vi "Teststand Edit STP.vi"(8 "error in":errorcluster, 10 "STP Data in":T1={"ECU CAN Port"="CAN1", "CMD"=130, "CAN Write Data"=[], "Response Decoder"=enum."String", "String"={"Start Index"=0, "Length"=-1}, "Number"={"MSB Index"=0, "LSB Index"=1}, "Boolean"={"Index"=0, "Bool"={"7"=FALSE, "6"=FALSE, "5"=FALSE, "4"=FALSE, "3"=FALSE, "2"=FALSE, "1"=FALSE, "0"=FALSE, "7 Enabled"=FALSE, "6 Enabled"=FALSE, "5 Enabled"=FALSE, "4 Enabled"=FALSE, "3 Enabled"=FALSE, "2 Enabled"=FALSE, "1 Enabled"=FALSE, "0 Enabled"=FALSE}}} {"CMD" items=["TSW_VERSION(130)"=130, "WAIT_EVENT(132)"=132, "SEQUENCER(133)"=133, "TSW_RESET(150)"=150, "CONFIG_ECU(151)"=151, "TEST_CORE (152)"=152, "TEST_WATCHDOG (153)"=153, "TEST_MONITORING (154)"=154, "READ_MEMORY (162)"=162, "WRITE_ERASE_MEMORY (164)"=164, "COMM_EXTERNAL (190)"=190, "COMM_INTERNAL (195)"=195, "GET_ANALOG_INPUT (210)"=210, "GET_DIGITAL_INPUT (211)"=211, "GET_FREQUENCY_INPUT (212)"=212, "TEST_INPUT_STRUCTURE (214)"=214, "GENERATE_OUTPUT_SIGNAL (220)"=220, "GENERATE_SYNCHRONIZED_OUTPUT_SIGNALS (221)"=221, "eDCU_Specific (250)"=250]; "CAN Write Data" format="%.0x"}, 11 "Sequence Context In":refnum<k7>) -> (0 "error out":errorcluster, 2 "STP Data out":T1={"ECU CAN Port"="CAN1", "CMD"=130, "CAN Write Data"=[], "Response Decoder"=enum."String", "String"={"Start Index"=0, "Length"=-1}, "Number"={"MSB Index"=0, "LSB Index"=1}, "Boolean"={"Index"=0, "Bool"={"7"=FALSE, "6"=FALSE, "5"=FALSE, "4"=FALSE, "3"=FALSE, "2"=FALSE, "1"=FALSE, "0"=FALSE, "7 Enabled"=FALSE, "6 Enabled"=FALSE, "5 Enabled"=FALSE, "4 Enabled"=FALSE, "3 Enabled"=FALSE, "2 Enabled"=FALSE, "1 Enabled"=FALSE, "0 Enabled"=FALSE}}} {"CMD" items=["TSW_VERSION(130)"=130, "WAIT_EVENT(132)"=132, "SEQUENCER(133)"=133, "TSW_RESET(150)"=150, "CONFIG_ECU(151)"=151, "TEST_CORE (152)"=152, "TEST_WATCHDOG (153)"=153, "TEST_MONITORING (154)"=154, "READ_MEMORY (162)"=162, "WRITE_ERASE_MEMORY (164)"=164, "COMM_EXTERNAL (190)"=190, "COMM_INTERNAL (195)"=195, "GET_ANALOG_INPUT (210)"=210, "GET_DIGITAL_INPUT (211)"=211, "GET_FREQUENCY_INPUT (212)"=212, "TEST_INPUT_STRUCTURE (214)"=214, "GENERATE_OUTPUT_SIGNAL (220)"=220, "GENERATE_SYNCHRONIZED_OUTPUT_SIGNALS (221)"=221, "eDCU_Specific (250)"=250]; "CAN Write Data" format="%.0x"})   [LabVIEW 2023, in "LTT_TeststandSteptypes.lvlib"]
uses:
  LTT_TeststandSteptypes.lvlib
  Control/STP Data.ctl
  HardwareAbstractionLayer_LVOOP/CAN/CAN Application Protocols/STP Protocol_class/Ctrls/STP CMD.ctl
  <vilib>/addons/TestStand/_TSUtility.llb/TestStand - Start Modal Dialog (Sequence Context).vi
  <vilib>/addons/TestStand/_TSUtility.llb/TestStand - End Modal Dialog (Sequence Context).vi
  HardwareAbstractionLayer_LVOOP/Database/Database.lvclass
  HardwareAbstractionLayer_LVOOP/Database/SQL Public VI/Control/DB Options.ctl
  HardwareAbstractionLayer_LVOOP/CAN/CAN Application Protocols/STP Protocol_class/STP Protocol.lvclass
panel:
  in  "Close":bool
  in  "OK":bool
  # "Help : the index will choose the one element in an array and compare its true or false"
  # "Bit"
  # "Value"
  # "Enabled"
  # "Help : if the LSB index is -1 then it will take only MSB value"
  # "Help : if length -1 then it will take the entire array"
  # "Help : the index will choose the one element in an array and compare its true or false"
  # "Bit"
  # "Value"
  # "Enabled"
  # "Help : if the LSB index is -1 then it will take only MSB value"
  # "Help : if length -1 then it will take the entire array"
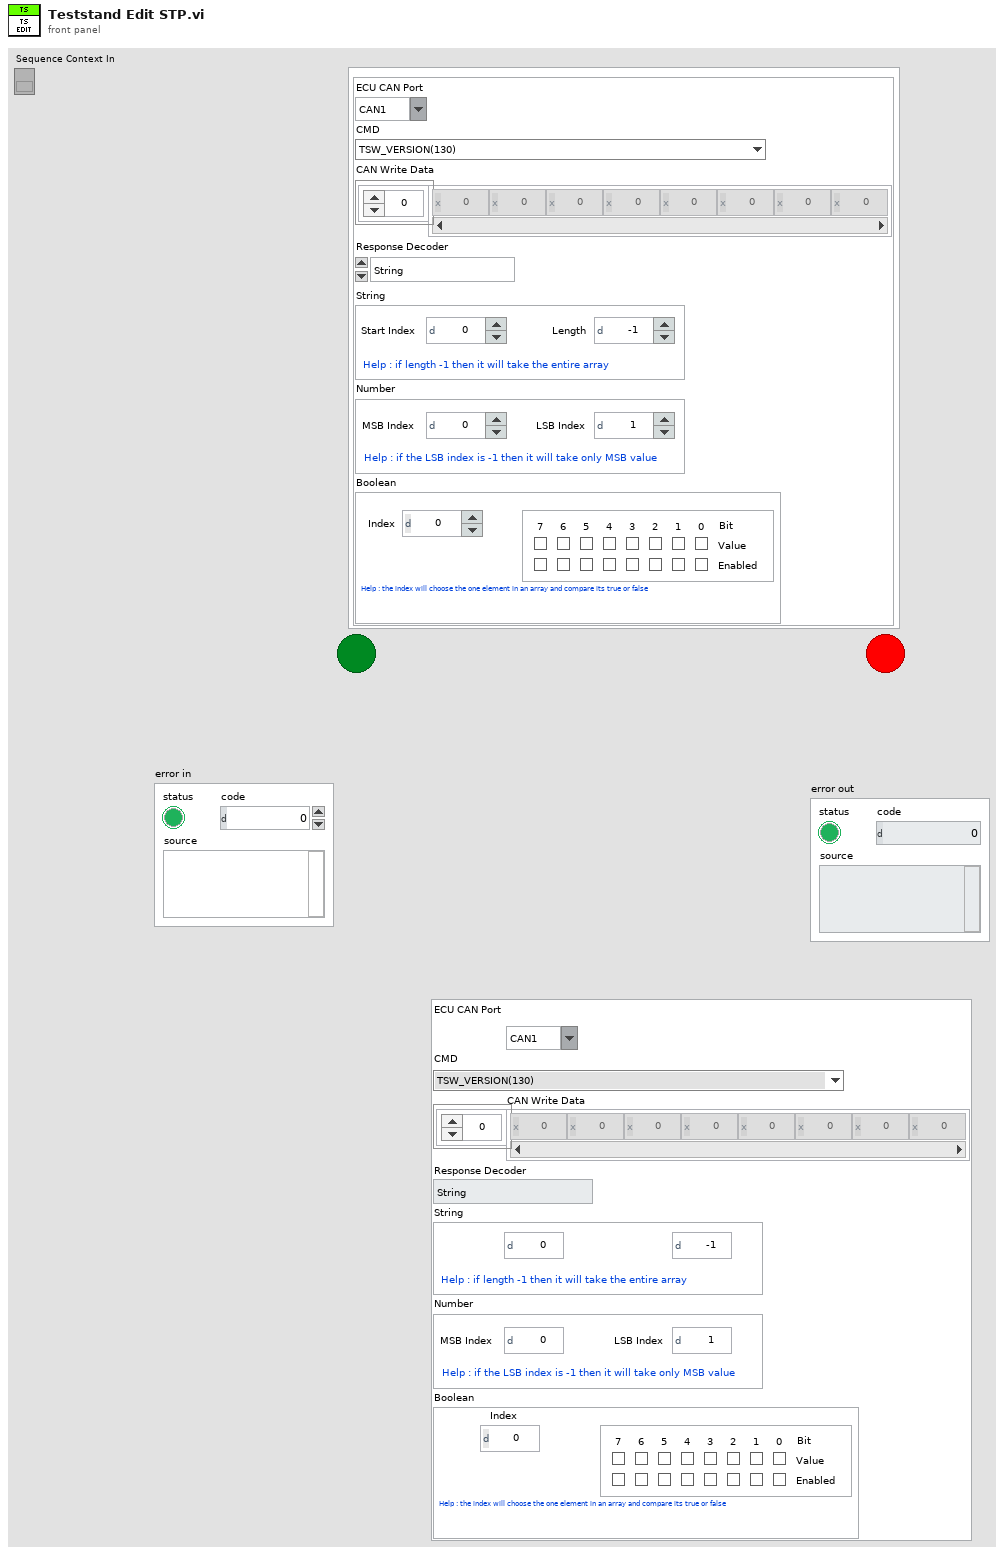
[diagram p1: front panel]
types:
  T1 = typedef "LTT_TeststandSteptypes.lvlib/STP Data.ctl" = cluster{"ECU CAN Port":string, "CMD":T2, "CAN Write Data":u8[], "Response Decoder":enum16{"String", "Number", "Boolean"}, "String":cluster{"Start Index":i32, "Length":i32}, "Number":cluster{"MSB Index":i32, "LSB Index":i32}, "Boolean":cluster{"Index":i32, "Bool":cluster{"7":bool, "6":bool, "5":bool, "4":bool, "3":bool, "2":bool, "1":bool, "0":bool, "7 Enabled":bool, "6 Enabled":bool, "5 Enabled":bool, "4 Enabled":bool, "3 Enabled":bool, "2 Enabled":bool, "1 Enabled":bool, "0 Enabled":bool}}}
  T2 = typedef "HardwareAbstractionLayer_LVOOP.lvlib/CAN Application Protocols Lib.lvlib/STP Protocol.lvclass/STP CMD.ctl" = u8
  T3 = typedef "HardwareAbstractionLayer_LVOOP.lvlib/Database.lvclass/DB Options.ctl" = enum16{"Init", "Select Data", "Insert Data", "Update Data", "Delete Data", "Execute Query", "Create Schema", "Create Table", "List Tables", "List Columns", "Close"}
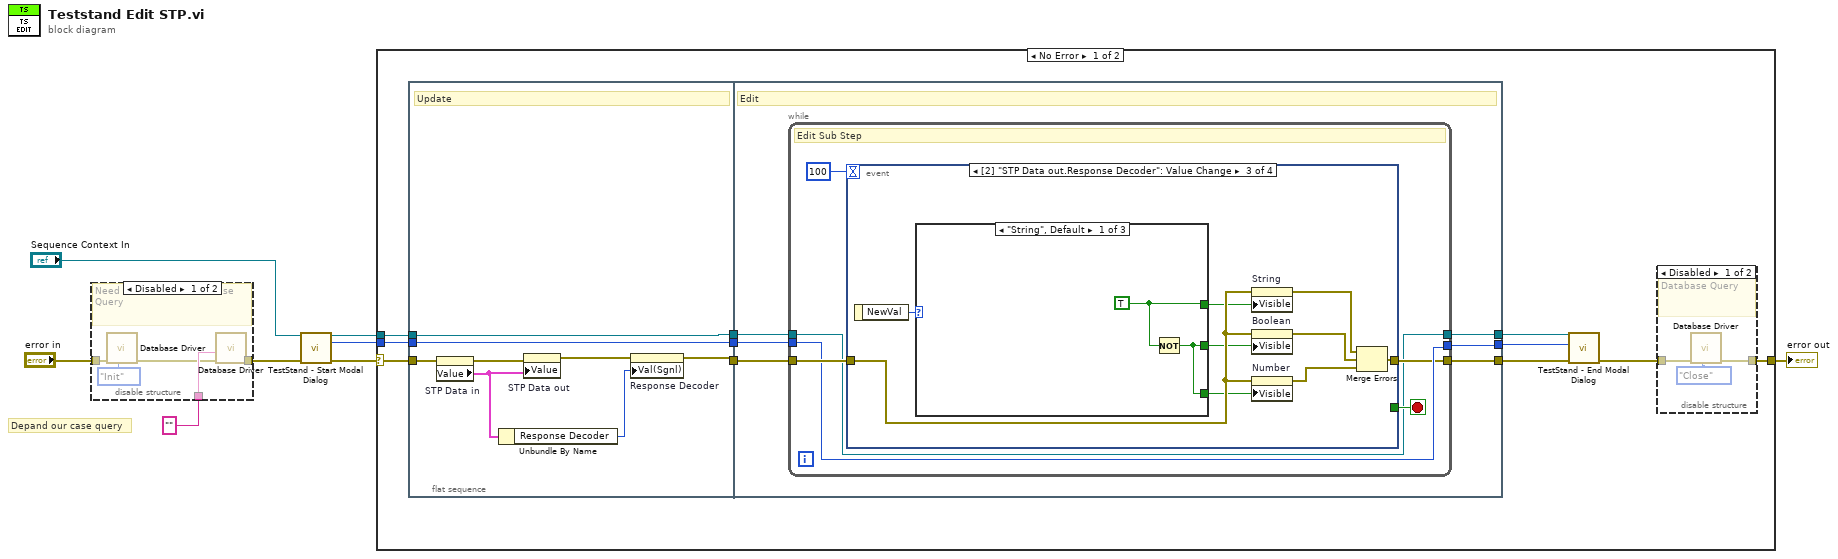
[diagram p0: block diagram]
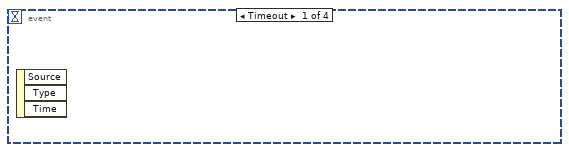
[diagram p3: hidden frame]
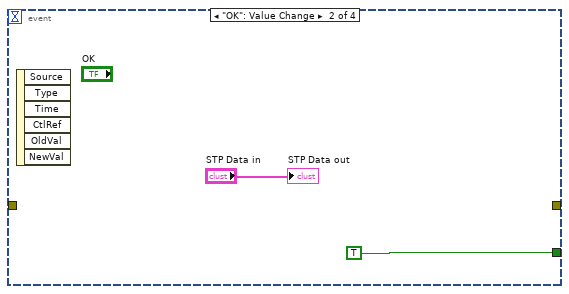
[diagram p4: hidden frame]
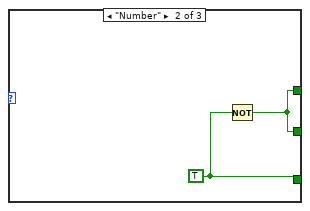
[diagram p5: hidden frame]
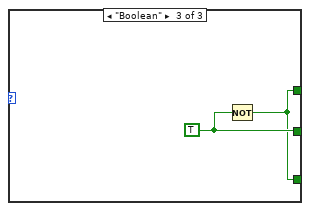
[diagram p6: hidden frame]
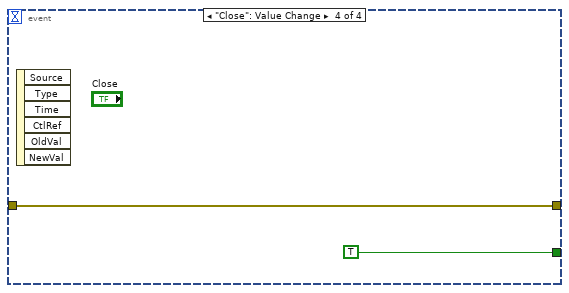
[diagram p7: hidden frame]
diagram:
  # "Depand our case query"
  n1 = disable-structure shown="Disabled" {
    disable-tunnel: "error in" -> [w13 _]
    disable-tunnel: [w12 _] -> w3
    disable-tunnel: "" ("SQL query") -> [w11 _]
    frame Disabled {
      # "Need to Enable for Database Query"
      n2 = call "Database Driver.vi"("Options"=DB_Options."Init", "error in"=w13) -> ("error out"=w10:errorcluster)  [unwired: 6 in, 3 out]
      n3 = call "Database Driver.vi"("error in"=w10, "SQL query"=w11) -> ("error out"=w12:errorcluster)  [unwired: 6 in, 3 out]
    }
    frame Enabled {
    }
  }
  n4 = call-poly <vilib>:"TestStand - Start Modal Dialog.vi"("Sequence Context In"="Sequence Context In", "error in (no error)"=w3) -> ("Sequence Context Out"=w5:refnum<k7>, "Modal ID"=w4:i32, "error out"=w6:errorcluster)  [unwired: 9 in, 2 out]
  n5 = case shown="No Error" w6 {
    selector: w6 -> [w21 w67]
    tunnel: w5 -> [w18 _]
    tunnel: w4 -> [w17 _]
    tunnel: [w15 w67] -> w1
    frame No Error {
      n6 = flat-sequence {
        tunnel: w21 -> [w33]
        tunnel: [w30] -> w24
        tunnel: w18 -> [w35]
        tunnel: w17 -> [w34]
        tunnel: [w35] -> w23
        tunnel: [w34] -> w22
        tunnel: w24 -> [w39]
        tunnel: [w37] -> w20
        tunnel: w23 -> [w41]
        tunnel: w22 -> [w40]
        tunnel: [w38] -> w16
        tunnel: [w36] -> w14
        frame #0 {
          # "Update"
          n7 = property on="STP Data in" class="Clust (strict)"(error in=w33) -> (error out=w32:errorcluster, "Value"=w29:T1)  [unwired: 1 in, 1 out]
          n8 = Unbundle By Name(w29) -> ("Response Decoder"=w28:enum16{"String", "Number", "Boolean"})
          n9 = property on="STP Data out" class="Clust (strict)"(error in=w32, "Value"=w29) -> (error out=w31:errorcluster)  [unwired: 1 in, 1 out]
          n10 = property on="Response Decoder" class="Enum (strict)"(error in=w31, "Val(Sgnl)"=w28) -> (error out=w30:errorcluster)  [unwired: 1 in, 1 out]
        }
        frame #1 {
          # "Edit"
          n11 = while {
            tunnel: w41 -> [w42]
            tunnel: w40 -> [w44]
            tunnel: w39 -> [w45]
            tunnel: [w44] -> w38
            tunnel: [w43] -> w37
            tunnel: [w42] -> w36
            stop <- w46 stop-if-true
            # "Edit Sub Step"
            n12 = event shown="[2] \"STP Data out.Response Decoder\": Value Change" {
              selector: _ -> [_ _ _ _]
              dyn-events: _ -> [_ _ _ _]
              timeout: 100 -> [_ _ _ _]
              tunnel: [_ TRUE _ TRUE] -> w46
              tunnel: w45 -> [_ _ w53 w65]
              tunnel: [_ _ w57 w65] -> w43
              event Timeout {
                n13 = event-data() -> ()  [unwired: 1 in, 3 out]
              }
              event "OK": Value Change {
                n14 = event-data() -> ()  [unwired: 1 in, 6 out]
                "STP Data out" <- "STP Data in"
              }
              event Value Change {
                n15 = event-data() -> ("NewVal"=w58:enum16{"String", "Number", "Boolean"})  [unwired: 1 in]
                n16 = case shown="\"String\", Default" w58 {
                  tunnel: [w60 w62 w63] -> w52
                  tunnel: [w59 w62 w64] -> w51
                  tunnel: [w59 w61 w63] -> w50
                  frame "String", Default {
                    w60 = TRUE
                    n17 = Not(x=w60) -> (.not. x?=w59:bool)
                  }
                  frame "Number" {
                    w61 = TRUE
                    n18 = Not(x=w61) -> (.not. x?=w62:bool)
                  }
                  frame "Boolean" {
                    w64 = TRUE
                    n19 = Not(x=w64) -> (.not. x?=w63:bool)
                  }
                }
                n20 = property on="String" class="Clust (strict)"(error in=w53, "Visible"=w52) -> (error out=w54:errorcluster)  [unwired: 1 in, 1 out]
                n21 = property on="Boolean" class="Clust (strict)"(error in=w53, "Visible"=w51) -> (error out=w55:errorcluster)  [unwired: 1 in, 1 out]
                n22 = property on="Number" class="Clust (strict)"(error in=w53, "Visible"=w50) -> (error out=w56:errorcluster)  [unwired: 1 in, 1 out]
                n23 = Merge Errors(w54, w55, w56) -> (w57:errorcluster)
              }
              event "Close": Value Change {
                n24 = event-data() -> ()  [unwired: 1 in, 6 out]
              }
            }
          }
        }
      }
      n25 = call-poly <vilib>:"TestStand - End Modal Dialog.vi"("Sequence Context In"=w14, "Modal ID"=w16, "error in (no error)"=w20) -> ("error out"=w19:errorcluster)  [unwired: 12 in]
      n26 = disable-structure shown="Disabled" {
        disable-tunnel: w19 -> [w27 _]
        disable-tunnel: [w26 _] -> w15
        frame Disabled {
          # "Need to Enable for Database Query"
          n27 = call "Database Driver.vi"("Options"=DB_Options."Close", "error in"=w27) -> ("error out"=w26:errorcluster)  [unwired: 6 in, 3 out]
        }
        frame Enabled {
        }
      }
    }
    frame Error {
    }
  }
  "error out" <- w1
